vi "ForwardKinematics3DOFChair.vi"(0 "theta2":dbl, 1 "theta1":dbl, 4 "L2":dbl, 5 "seat":dbl, 6 "theta3":dbl, 7 "back":dbl, 11 "L1":dbl) -> (10 "x3":dbl, 12 "y4":dbl, 13 "y2":dbl, 14 "x1":dbl, 15 "y1":dbl, 17 "x4":dbl, 18 "x2":dbl, 19 "y3":dbl)   [LabVIEW 2024]
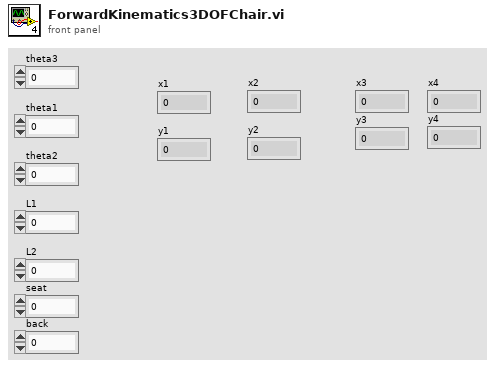
[diagram p1: front panel]
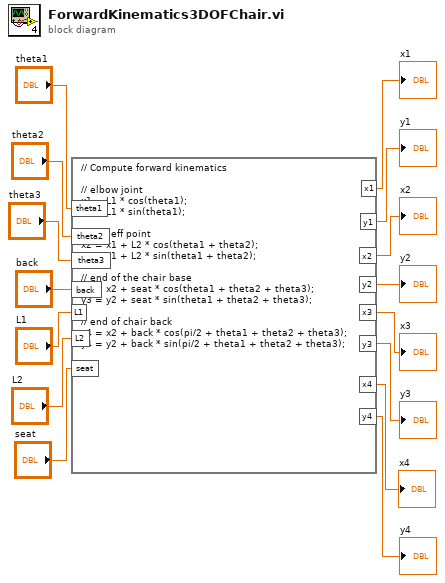
[diagram p0: block diagram]
diagram:
  n1 = formula code="// Compute forward kinematics\n\n// elbow joint\nx1 = L1 * cos(theta1);\ny1 = L1 * sin(theta1);\n\n// end eff point\nx2 = x1 + L2 * cos(theta1 + theta2);\ny2 = y1 + L2 * sin(theta1 + theta2);\n\n// end of the chair base\nx3 = x2 + seat * cos(theta1 + theta2 + theta3);\ny3 = y2 + seat * sin(theta1 + theta2 + theta3);\n\n// end of chair back\nx4 = x2 + back * cos(pi/2 + theta1 + theta2 + theta3);\ny4 = y2 + back * sin(pi/2 + theta1 + theta2 + theta3);"("theta1"="theta1", "theta2"="theta2", "L1"="L1", "L2"="L2", "theta3"="theta3", "seat"="seat", "back"="back") -> ("x1"=→"x1":dbl, "y1"=→"y1":dbl, "x2"=→"x2":dbl, "y2"=→"y2":dbl, "y3"=→"y3":dbl, "x3"=→"x3":dbl, "x4"=→"x4":dbl, "y4"=→"y4":dbl)
